vi "Service to micros.vi"(8 "error in (no error)":errorcluster, 10 "Caracter":string, 11 "User Interface in":refnum<class "User Interface.lvclass">) -> (0 "error out":errorcluster, 3 "User Interface out":refnum<class "User Interface.lvclass">)   [LabVIEW 2020, in "User Interface.lvlib" / "User Interface.lvclass"]
uses:
  User Interface.lvclass
  User Interface.lvclass/User Interface.ctl
  Hardware/Hardware Messages/Sequence Micro Msg/Sequence Micro Msg.lvclass/Sequence Micro Msg.ctl
  <vilib>/ActorFramework/Message Enqueuer/Message Enqueuer.lvclass/Message Enqueuer.ctl
  <vilib>/ActorFramework/Message Enqueuer/Enqueue.vi
  Hardware/Hardware Messages/Sequence Micro Msg/Sequence Micro Msg.lvclass
  C:/Program Files (x86)/National Instruments/LabVIEW 2020/vi.lib/ActorFramework/Message/Message.lvclass
  <vilib>/ActorFramework/Message Priority Queue/Priority Enqueue.vi
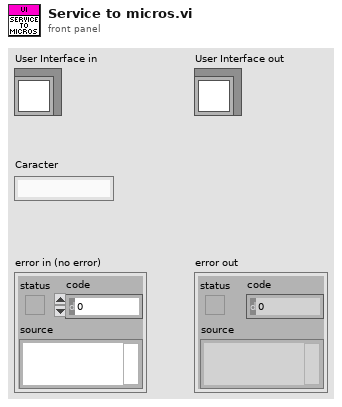
[diagram p1: front panel]
types:
  T1 = cluster{"Water Presure":bool, "Soap":bool, "Water Wash":bool, "Dry":bool, "Vacuum Cleaner":bool, "Motor Wash":bool, "Wax":bool}
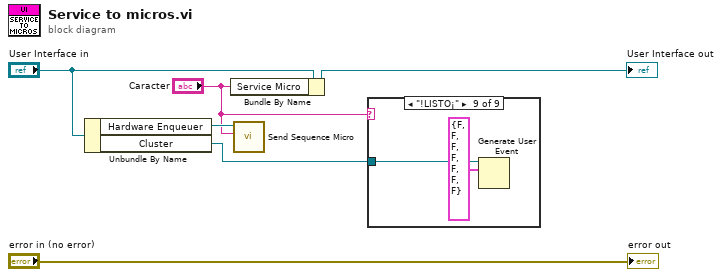
[diagram p0: block diagram]
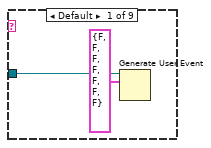
[diagram p2: hidden frame]
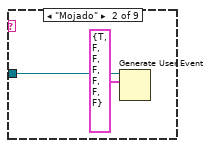
[diagram p3: hidden frame]
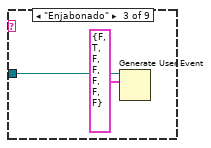
[diagram p4: hidden frame]
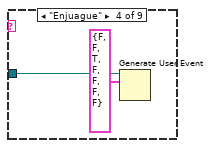
[diagram p5: hidden frame]
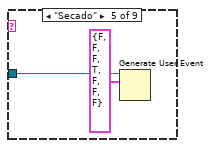
[diagram p6: hidden frame]
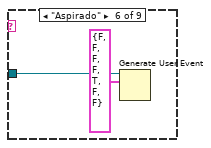
[diagram p7: hidden frame]
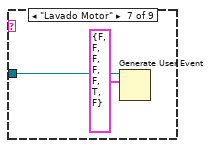
[diagram p8: hidden frame]
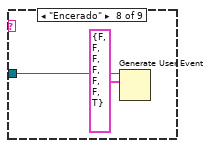
[diagram p9: hidden frame]
diagram:
  n1 = Unbundle By Name("User Interface in") -> ("Hardware Enqueuer"=w3:refnum<class "Message Enqueuer.lvclass">, "Cluster"=w1:refnum<user-event>)
  n2 = Bundle By Name(cluster="User Interface in", "Service Micro"="Caracter") -> (→"User Interface out":refnum<class "User Interface.lvclass">)
  n3 = call "Send Sequence Micro.vi"("Status"="Caracter", "Message Enqueuer"=w3) -> ()  [unwired: 8 in, 2 out]
  n4 = case shown="\"!LISTO¡\"" "Caracter" {
    tunnel: w1 -> [w8 w10 w12 w14 w16 w18 w20 w22 w24]
    frame Default {
      n5 = Generate User Event(user event=w8, event data cluster=T1 {"Water Presure"=FALSE, "Soap"=FALSE, "Water Wash"=FALSE, "Dry"=FALSE, "Vacuum Cleaner"=FALSE, "Motor Wash"=FALSE, "Wax"=FALSE} ("event data")) -> ()  [unwired: 2 in, 2 out]
    }
    frame "Mojado" {
      n6 = Generate User Event(user event=w10, event data cluster=T1 {"Water Presure"=TRUE, "Soap"=FALSE, "Water Wash"=FALSE, "Dry"=FALSE, "Vacuum Cleaner"=FALSE, "Motor Wash"=FALSE, "Wax"=FALSE} ("event data")) -> ()  [unwired: 2 in, 2 out]
    }
    frame "Enjabonado" {
      n7 = Generate User Event(user event=w12, event data cluster=T1 {"Water Presure"=FALSE, "Soap"=TRUE, "Water Wash"=FALSE, "Dry"=FALSE, "Vacuum Cleaner"=FALSE, "Motor Wash"=FALSE, "Wax"=FALSE} ("event data")) -> ()  [unwired: 2 in, 2 out]
    }
    frame "Enjuague" {
      n8 = Generate User Event(user event=w14, event data cluster=T1 {"Water Presure"=FALSE, "Soap"=FALSE, "Water Wash"=TRUE, "Dry"=FALSE, "Vacuum Cleaner"=FALSE, "Motor Wash"=FALSE, "Wax"=FALSE} ("event data")) -> ()  [unwired: 2 in, 2 out]
    }
    frame "Secado" {
      n9 = Generate User Event(user event=w16, event data cluster=T1 {"Water Presure"=FALSE, "Soap"=FALSE, "Water Wash"=FALSE, "Dry"=TRUE, "Vacuum Cleaner"=FALSE, "Motor Wash"=FALSE, "Wax"=FALSE} ("event data")) -> ()  [unwired: 2 in, 2 out]
    }
    frame "Aspirado" {
      n10 = Generate User Event(user event=w18, event data cluster=T1 {"Water Presure"=FALSE, "Soap"=FALSE, "Water Wash"=FALSE, "Dry"=FALSE, "Vacuum Cleaner"=TRUE, "Motor Wash"=FALSE, "Wax"=FALSE} ("event data")) -> ()  [unwired: 2 in, 2 out]
    }
    frame "Lavado Motor" {
      n11 = Generate User Event(user event=w20, event data cluster=T1 {"Water Presure"=FALSE, "Soap"=FALSE, "Water Wash"=FALSE, "Dry"=FALSE, "Vacuum Cleaner"=FALSE, "Motor Wash"=TRUE, "Wax"=FALSE} ("event data")) -> ()  [unwired: 2 in, 2 out]
    }
    frame "Encerado" {
      n12 = Generate User Event(user event=w22, event data cluster=T1 {"Water Presure"=FALSE, "Soap"=FALSE, "Water Wash"=FALSE, "Dry"=FALSE, "Vacuum Cleaner"=FALSE, "Motor Wash"=FALSE, "Wax"=TRUE} ("event data")) -> ()  [unwired: 2 in, 2 out]
    }
    frame "!LISTO¡" {
      n13 = Generate User Event(user event=w24, event data cluster=T1 {"Water Presure"=FALSE, "Soap"=FALSE, "Water Wash"=FALSE, "Dry"=FALSE, "Vacuum Cleaner"=FALSE, "Motor Wash"=FALSE, "Wax"=FALSE} ("event data")) -> ()  [unwired: 2 in, 2 out]
    }
  }
  "error out" <- "error in (no error)"
